vi "ChangeLight.vi"(0 "object in":refnum<class "GreenState.lvclass">, 5 "Error In":errorcluster) -> (14 "object out":refnum<class "State.lvclass">, 19 "Error Out":errorcluster)   [LabVIEW 2024, in "GreenState.lvclass"]
uses:
  GreenState.lvclass
  C:/Users/burakkorkmaz/Desktop/Leveling/labview-desing-patterns/State Pattern/State_interface/State.lvclass
  State_interface/State.lvclass
  RedState_class/RedState.lvclass
  GreenState.lvclass/GreenState.ctl
panel:
  # "Connector Pane"
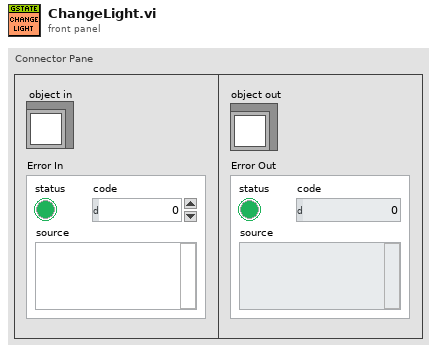
[diagram p1: front panel]
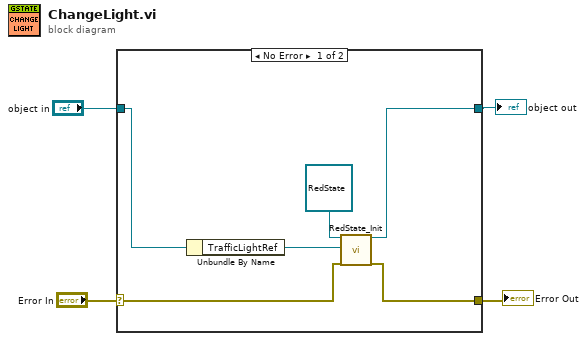
[diagram p0: block diagram]
diagram:
  n1 = case shown="No Error" "Error In" {
    selector: "Error In" -> [w7 w12]
    tunnel: [w6 w12] -> w3
    tunnel: [w5 w11] -> w1
    tunnel: "object in" -> [w10 w11]
    frame No Error {
      n2 = Unbundle By Name(w10) -> ("TrafficLightRef"=w8:refnum<class "TrafficLight.lvclass">)
      n3 = call "RedState_Init.vi"("object in"=refnum<class "RedState.lvclass"> refnum ("RedState"), "TrafficLight"=w8, "Error In"=w7) -> ("object out"=w5:refnum<class "RedState.lvclass">, "Error Out"=w6:errorcluster)  [unwired: 15 in]
    }
    frame Error {
    }
  }
  "Error Out" <- w3
  "object out" <- w1
